vi "Measurement6DoFToJSON.vi"(6 "Comment":string, 8 "ErrorIn":errorcluster, 9 "GyroData":waveform(dbl)[](array[waveform]), 10 "AccelData":waveform(dbl)[](array[waveform]), 11 "JSONIn":refnum<class "JSON Object.lvclass">) -> (0 "ErrorOut":errorcluster, 2 "JSONMeasurement6DoF":string, 3 "JSONOut":refnum<class "JSON Object.lvclass">)   [LabVIEW 2016]
uses:
  <vilib>/addons/JSON API/JSON Object/JSON Object.lvclass
  D:/Programy/National Instruments/LabVIEW 2016/vi.lib/addons/JSON API/JSON Value/JSON Value.lvclass
  JSONStreamType.ctl
  <vilib>/addons/JSON API/JSON Object/Set Object Item by name.vi
  <vilib>/addons/JSON API/JSON Scalar/JSON Scalar.lvclass
  <vilib>/addons/JSON API/JSON Array/JSON Array.lvclass
  <vilib>/addons/JSON API/JSON Scalar/Set DBL.vi
  <vilib>/addons/JSON API/JSON Scalar/Set String.vi
  <vilib>/addons/JSON API/JSON Array/Set JSON Array.vi
  <vilib>/addons/JSON API/JSON Value/Get as JSON string (pretty).vi
  <vilib>/addons/JSON API/Get Polymorphic/JSON GetSet.lvlib
  <vilib>/addons/JSON API/JSON Value/JSON Value.lvclass
panel:
  in  "StreamType(Raw)":T1
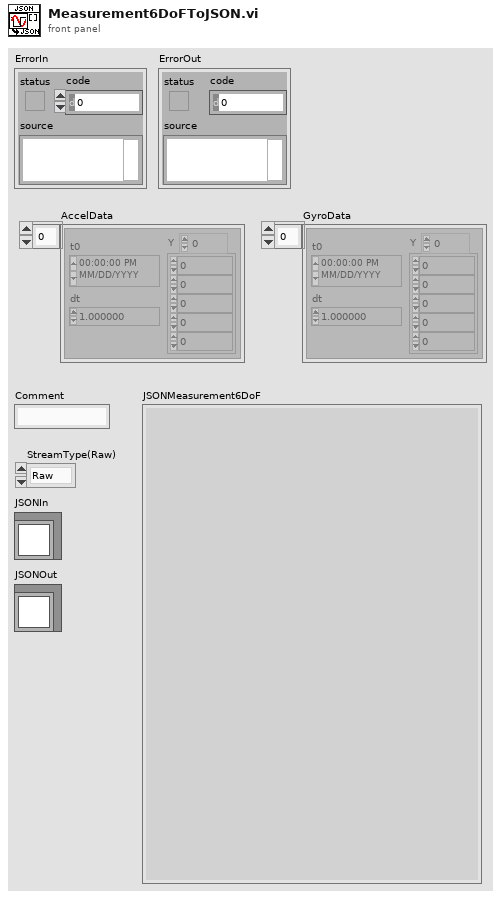
[diagram p1: front panel]
types:
  T1 = typedef "JSONStreamType.ctl" = enum16{"Raw", "Pretty"}
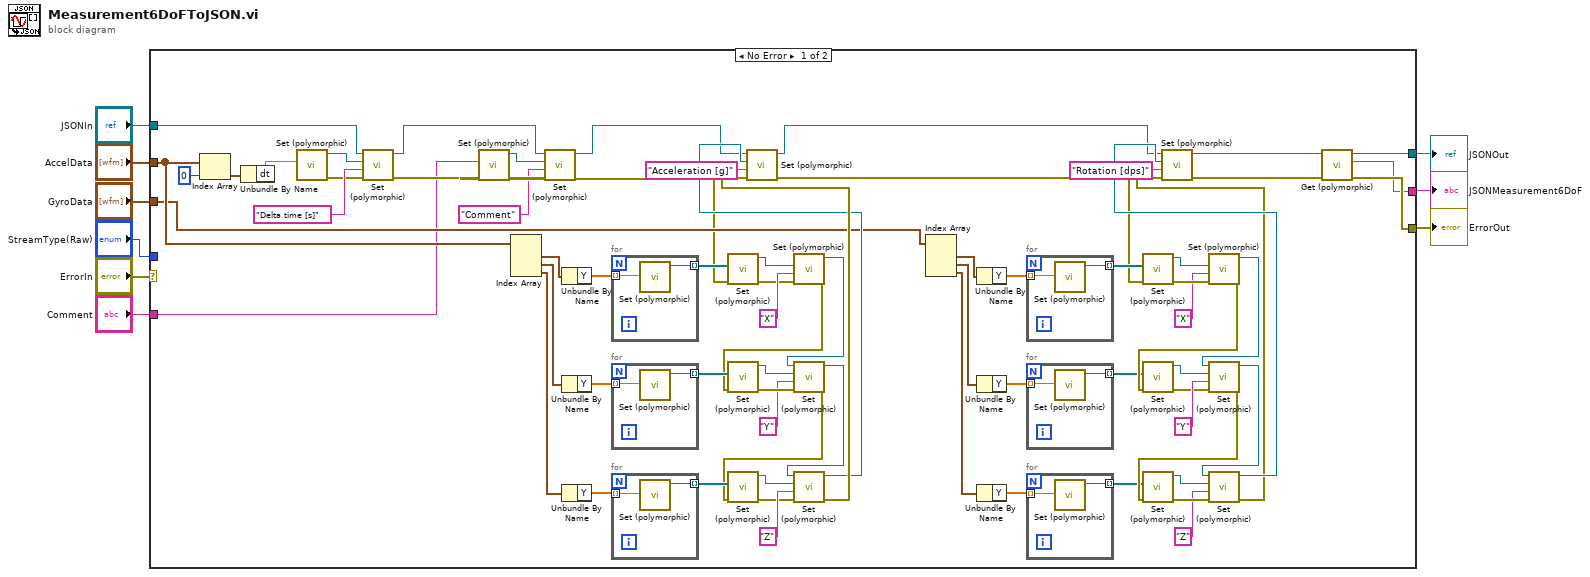
[diagram p0: block diagram]
diagram:
  n1 = case shown="No Error" "ErrorIn" {
    selector: "ErrorIn" -> [_ w96]
    tunnel: [w20 w96] -> w8
    tunnel: "JSONIn" -> [w82 w95]
    tunnel: "AccelData" -> [w79 _]
    tunnel: "GyroData" -> [w22 _]
    tunnel: "StreamType(Raw)" -> [_ _]
    tunnel: [w19 _] -> w3
    tunnel: [w18 w95] -> w2
    tunnel: "Comment" -> [w10 _]
    frame No Error {
      n2 = Index Array(array=w79, index=0) -> (element=w77:waveform(dbl))
      n3 = Unbundle By Name(w77) -> ("dt"=w76:dbl)
      n4 = call-poly <vilib>:"Set (polymorphic).vi"("Numeric"=w76) -> ("error out"=w74:errorcluster, "JSON Scalar out"=w81:refnum<class "JSON Scalar.lvclass">)  [unwired: 9 in]
      n5 = call-poly <vilib>:"Set (polymorphic).vi"("error in (no error)"=w74, "name"="Delta time [s]", "Value"=w81, "JSON Object in"=w82) -> ("error out"=w16:errorcluster, "JSON Object out"=w14:refnum<class "JSON Object.lvclass">)  [unwired: 5 in, 1 out]
      n6 = call-poly <vilib>:"Set (polymorphic).vi"("error in (no error)"=w16, "String"=w10) -> ("error out"=w15:errorcluster, "JSON Scalar out"=w12:refnum<class "JSON Scalar.lvclass">)  [unwired: 8 in]
      n7 = Index Array(array=w79) -> (element #1=w75:waveform(dbl), element #2=w72:waveform(dbl), element #3=w71:waveform(dbl))  [unwired: 3 in]
      n8 = call-poly <vilib>:"Set (polymorphic).vi"("error in (no error)"=w15, "name"="Comment", "Value"=w12, "JSON Object in"=w14) -> ("error out"=w17:errorcluster, "JSON Object out"=w13:refnum<class "JSON Object.lvclass">)  [unwired: 5 in, 1 out]
      n9 = Unbundle By Name(w75) -> ("Y"=w67:dbl[])
      n10 = Unbundle By Name(w72) -> ("Y"=w56:dbl[])
      n11 = Unbundle By Name(w71) -> ("Y"=w57:dbl[])
      n12 = for {
        tunnel: w67 -> [w94] mode=indexing
        tunnel: [w93] -> w66 mode=indexing
        n13 = call-poly <vilib>:"Set (polymorphic).vi"("Numeric"=w94) -> ("JSON Scalar out"=w93:refnum<class "JSON Scalar.lvclass">)  [unwired: 9 in, 1 out]
      }
      n14 = for {
        tunnel: w56 -> [w92] mode=indexing
        tunnel: [w91] -> w65 mode=indexing
        n15 = call-poly <vilib>:"Set (polymorphic).vi"("Numeric"=w92) -> ("JSON Scalar out"=w91:refnum<class "JSON Scalar.lvclass">)  [unwired: 9 in, 1 out]
      }
      n16 = for {
        tunnel: w57 -> [w90] mode=indexing
        tunnel: [w89] -> w58 mode=indexing
        n17 = call-poly <vilib>:"Set (polymorphic).vi"("Numeric"=w90) -> ("JSON Scalar out"=w89:refnum<class "JSON Scalar.lvclass">)  [unwired: 9 in, 1 out]
      }
      n18 = call-poly <vilib>:"Set (polymorphic).vi"("error in (no error)"=w17, "Array"=w66) -> ("error out"=w69:errorcluster, "JSON Array out"=w68:refnum<class "JSON Array.lvclass">)  [unwired: 8 in]
      n19 = call-poly <vilib>:"Set (polymorphic).vi"("error in (no error)"=w69, "name"="X", "Value"=w68) -> ("error out"=w53:errorcluster, "JSON Object out"=w55:refnum<class "JSON Object.lvclass">)  [unwired: 6 in, 1 out]
      n20 = call-poly <vilib>:"Set (polymorphic).vi"("error in (no error)"=w53, "Array"=w65) -> ("error out"=w63:errorcluster, "JSON Array out"=w64:refnum<class "JSON Array.lvclass">)  [unwired: 8 in]
      n21 = call-poly <vilib>:"Set (polymorphic).vi"("error in (no error)"=w63, "name"="Y", "Value"=w64, "JSON Object in"=w55) -> ("error out"=w52:errorcluster, "JSON Object out"=w54:refnum<class "JSON Object.lvclass">)  [unwired: 5 in, 1 out]
      n22 = call-poly <vilib>:"Set (polymorphic).vi"("error in (no error)"=w52, "Array"=w58) -> ("error out"=w60:errorcluster, "JSON Array out"=w59:refnum<class "JSON Array.lvclass">)  [unwired: 8 in]
      n23 = call-poly <vilib>:"Set (polymorphic).vi"("error in (no error)"=w60, "name"="Z", "Value"=w59, "JSON Object in"=w54) -> ("error out"=w51:errorcluster, "JSON Object out"=w50:refnum<class "JSON Object.lvclass">)  [unwired: 5 in, 1 out]
      n24 = call-poly <vilib>:"Set (polymorphic).vi"("error in (no error)"=w51, "name"="Acceleration [g]", "Value"=w50, "JSON Object in"=w13) -> ("error out"=w23:errorcluster, "JSON Object out"=w24:refnum<class "JSON Object.lvclass">)  [unwired: 5 in, 1 out]
      n25 = Index Array(array=w22) -> (element #1=w25:waveform(dbl), element #2=w27:waveform(dbl), element #3=w28:waveform(dbl))  [unwired: 3 in]
      n26 = Unbundle By Name(w25) -> ("Y"=w32:dbl[])
      n27 = Unbundle By Name(w27) -> ("Y"=w43:dbl[])
      n28 = Unbundle By Name(w28) -> ("Y"=w42:dbl[])
      n29 = for {
        tunnel: w32 -> [w88] mode=indexing
        tunnel: [w87] -> w33 mode=indexing
        n30 = call-poly <vilib>:"Set (polymorphic).vi"("Numeric"=w88) -> ("JSON Scalar out"=w87:refnum<class "JSON Scalar.lvclass">)  [unwired: 9 in, 1 out]
      }
      n31 = for {
        tunnel: w43 -> [w86] mode=indexing
        tunnel: [w85] -> w34 mode=indexing
        n32 = call-poly <vilib>:"Set (polymorphic).vi"("Numeric"=w86) -> ("JSON Scalar out"=w85:refnum<class "JSON Scalar.lvclass">)  [unwired: 9 in, 1 out]
      }
      n33 = for {
        tunnel: w42 -> [w84] mode=indexing
        tunnel: [w83] -> w41 mode=indexing
        n34 = call-poly <vilib>:"Set (polymorphic).vi"("Numeric"=w84) -> ("JSON Scalar out"=w83:refnum<class "JSON Scalar.lvclass">)  [unwired: 9 in, 1 out]
      }
      n35 = call-poly <vilib>:"Set (polymorphic).vi"("error in (no error)"=w23, "Array"=w33) -> ("error out"=w30:errorcluster, "JSON Array out"=w31:refnum<class "JSON Array.lvclass">)  [unwired: 8 in]
      n36 = call-poly <vilib>:"Set (polymorphic).vi"("error in (no error)"=w30, "name"="X", "Value"=w31) -> ("error out"=w46:errorcluster, "JSON Object out"=w44:refnum<class "JSON Object.lvclass">)  [unwired: 6 in, 1 out]
      n37 = call-poly <vilib>:"Set (polymorphic).vi"("error in (no error)"=w46, "Array"=w34) -> ("error out"=w36:errorcluster, "JSON Array out"=w35:refnum<class "JSON Array.lvclass">)  [unwired: 8 in]
      n38 = call-poly <vilib>:"Set (polymorphic).vi"("error in (no error)"=w36, "name"="Y", "Value"=w35, "JSON Object in"=w44) -> ("error out"=w47:errorcluster, "JSON Object out"=w45:refnum<class "JSON Object.lvclass">)  [unwired: 5 in, 1 out]
      n39 = call-poly <vilib>:"Set (polymorphic).vi"("error in (no error)"=w47, "Array"=w41) -> ("error out"=w39:errorcluster, "JSON Array out"=w40:refnum<class "JSON Array.lvclass">)  [unwired: 8 in]
      n40 = call-poly <vilib>:"Set (polymorphic).vi"("error in (no error)"=w39, "name"="Z", "Value"=w40, "JSON Object in"=w45) -> ("error out"=w48:errorcluster, "JSON Object out"=w49:refnum<class "JSON Object.lvclass">)  [unwired: 5 in, 1 out]
      n41 = call-poly <vilib>:"Set (polymorphic).vi"("error in (no error)"=w48, "name"="Rotation [dps]", "Value"=w49, "JSON Object in"=w24) -> ("error out"=w21:errorcluster, "JSON Object out"=w18:refnum<class "JSON Object.lvclass">)  [unwired: 5 in, 1 out]
      n42 = call-poly <vilib>:"Get (polymorphic).vi"("error in (no error)"=w21, "JSON Value in"=w18) -> ("error out"=w20:errorcluster, "<JSON>"=w19:string)  [unwired: 8 in]
    }
    frame Error {
    }
  }
  "ErrorOut" <- w8
  "JSONMeasurement6DoF" <- w3
  "JSONOut" <- w2
